vi "StartRunningNamedProtocol.vi"(10 "protocol name":string) -> ()   [LabVIEW 2018]
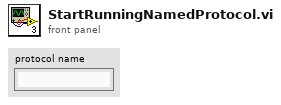
[diagram p1: front panel]
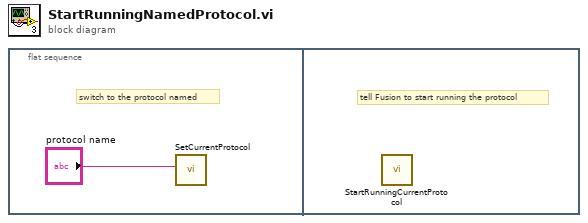
[diagram p0: block diagram]
diagram:
  n1 = flat-sequence {
    frame #0 {
      # "switch to the protocol named"
      n2 = call "SetCurrentProtocol.vi"("protocol name"="protocol name") -> ()  [unwired: 11 in]
    }
    frame #1 {
      # "tell Fusion to start running the protocol"
      n3 = call "StartRunningCurrentProtocol.vi"() -> ()  [unwired: 12 in]
    }
  }
